vi "Obtain Message Queue - Controller.vi"(8 "error in (no error)":errorcluster) -> (0 "error out":errorcluster, 3 "Controller":refnum<queue>)   [LabVIEW 2017, in "Message Queue.lvlib"]
doc: "Create a queue with the Message Cluster data type."
uses:
  Message Queue.lvlib
  Elevator/Controls/Elevator Command Event.ctl
  Elevator/Controls/Elevator Commands.ctl
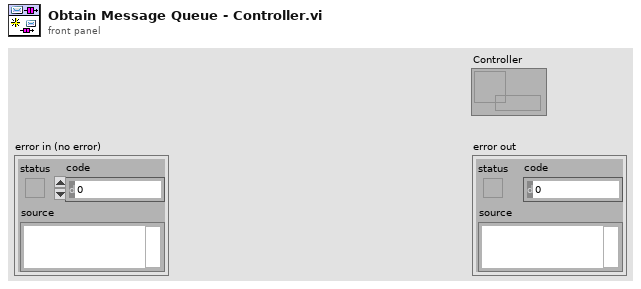
[diagram p1: front panel]
types:
  T1 = typedef "Elevator Command Event.ctl" = cluster{"Elevator Commands":T2, "Variant":variant}
  T2 = typedef "Elevator Commands.ctl" = enum16{"Go Up", "Go Down", "Go to Floor", "Emergency", "Open Doors", "Close Doors", "Start Move", "Move", "Finish Move", "Analysis"}
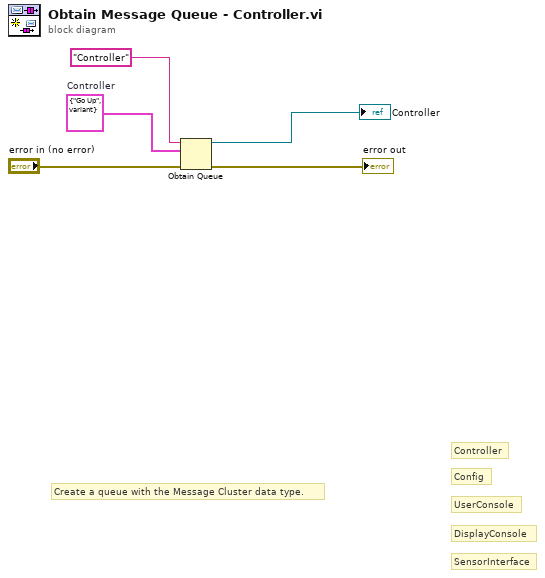
[diagram p0: block diagram]
diagram:
  w3 = T1 {"Elevator Commands"=enum."Go Up", "Variant"=variant}  # Controller
  # "SensorInterface"
  # "DisplayConsole"
  # "UserConsole"
  # "Config"
  # "Controller"
  # "Create a queue with the Message Cluster data type."
  n1 = Obtain Queue(name (unnamed)="Controller", element data type=w3, error in (no error)="error in (no error)") -> (queue out=→"Controller":refnum<queue>, error out=→"error out":errorcluster)  [unwired: 2 in, 1 out]
